vi "SendUpstreamMessage.vi"(8 "error in (no error)":errorcluster, 10 "UpstreamMsg":refnum<class "UpstreamMsgParent.lvclass">, 11 "ServiceManager in":refnum<class "ServiceManager.lvclass">) -> (0 "error out":errorcluster, 3 "ServiceManager out":refnum<class "ServiceManager.lvclass">)   [LabVIEW 2020, in "ServiceManager.lvlib" / "ServiceManager.lvclass"]
uses:
  ServiceManager.lvclass
  UpstreamMsg/UpstreamMsgParent/UpstreamMsgParent.lvclass
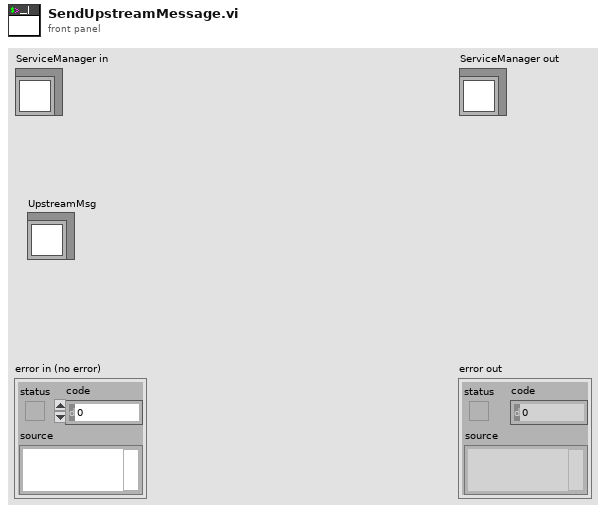
[diagram p1: front panel]
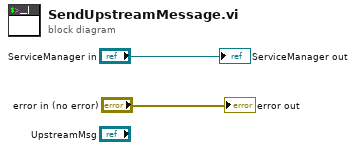
[diagram p0: block diagram]
diagram:
  "error out" <- "error in (no error)"
  "ServiceManager out" <- "ServiceManager in"
